vi "main.vi"() -> ()   [LabVIEW 2014]
uses:
  E:/labview_all/LabVIEW 2014/examples/Design Patterns/State Machine/support/State Machine Fundamentals - State Enum.ctl
  <vilib>/myRIO/Common/Instrument Driver Framework/myRIO v1.0/UART/vis/myRIO v1.0 Close UART.vi
  <vilib>/myRIO/Common/Instrument Driver Framework/Utilities/vis/FPGA Ref Manager.vi
  <vilib>/myRIO/Common/Instrument Driver Framework/myRIO v1.0/myRIO v1.0 Reset FPGA.vi
  <vilib>/myRIO/Common/Instrument Driver Framework/myRIO v1.0/IRQ/vis/myRIO v1.0 IRQ Info FGV.vi
  <vilib>/myRIO/Common/Instrument Driver Framework/myRIO v1.0/IRQ/vis/myRIO v1.0 Timer IRQ Info FGV.vi
  <vilib>/myRIO/Common/Instrument Driver Framework/myRIO v1.0/IRQ/vis/myRIO v1.0 ISR Agent.vi
  <vilib>/myRIO/Instrument Drivers/Utilities/Utilities.lvlib
panel:
  in  "布尔":bool
  out "y1 2":i32
  out "y1":i32
  out "shuzhi":dbl
  out "shuiping":dbl
  out "采集速度":bool
  out "state":T1
  in  "车速控制":dbl(slide) scale=-1.0..1.0
  in  "舵机":dbl(slide) min=-100.0 max=100.0 scale=-200.0..200.0
  out "Right（0）":bool
  out "Left（1）":bool
  out "四个角点":i32[][](array[numeric])
  in  "停止":bool
  out "Image":T2(plugin-control)
  # "X"
  # "Y"
  # "X"
  # "Y"
  # "左下"
  # "左上"
  # "右下"
  # "右上"
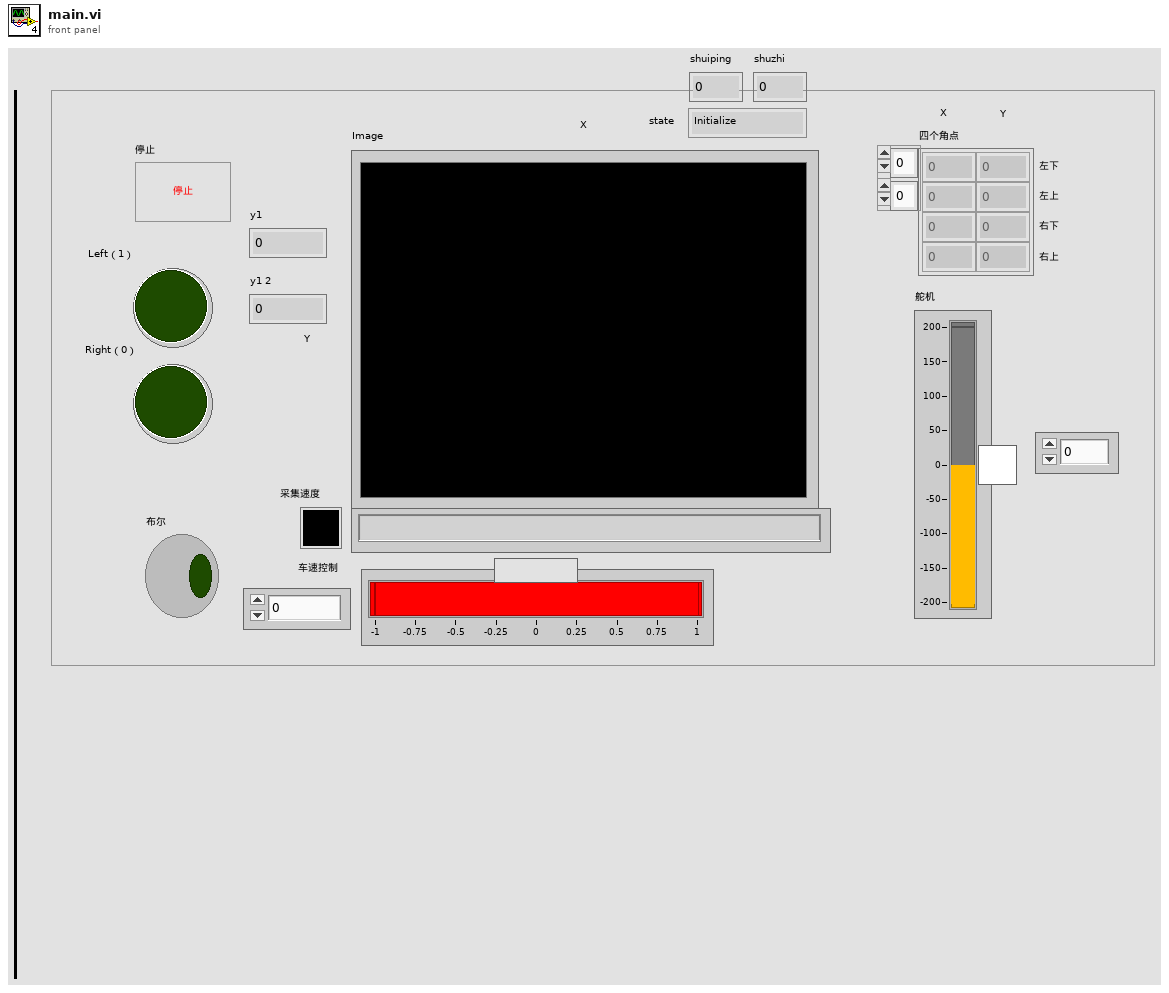
[diagram p1: front panel]
types:
  T1 = typedef "State Machine Fundamentals - State Enum.ctl" = enum16{"Initialize", "L or R", "L1", "L2", "R1", "R2", "IN", "STOP"}
  T2 = typedef "IMAQ Image.ctl" = refnum<image>
  T3 = cluster{"Optional Rectangle[0]":i32, "Optional Rectangle[1]":i32, "Optional Rectangle[2]":i32, "Optional Rectangle[3]":i32, "Optional Rectangle[4]":i32}
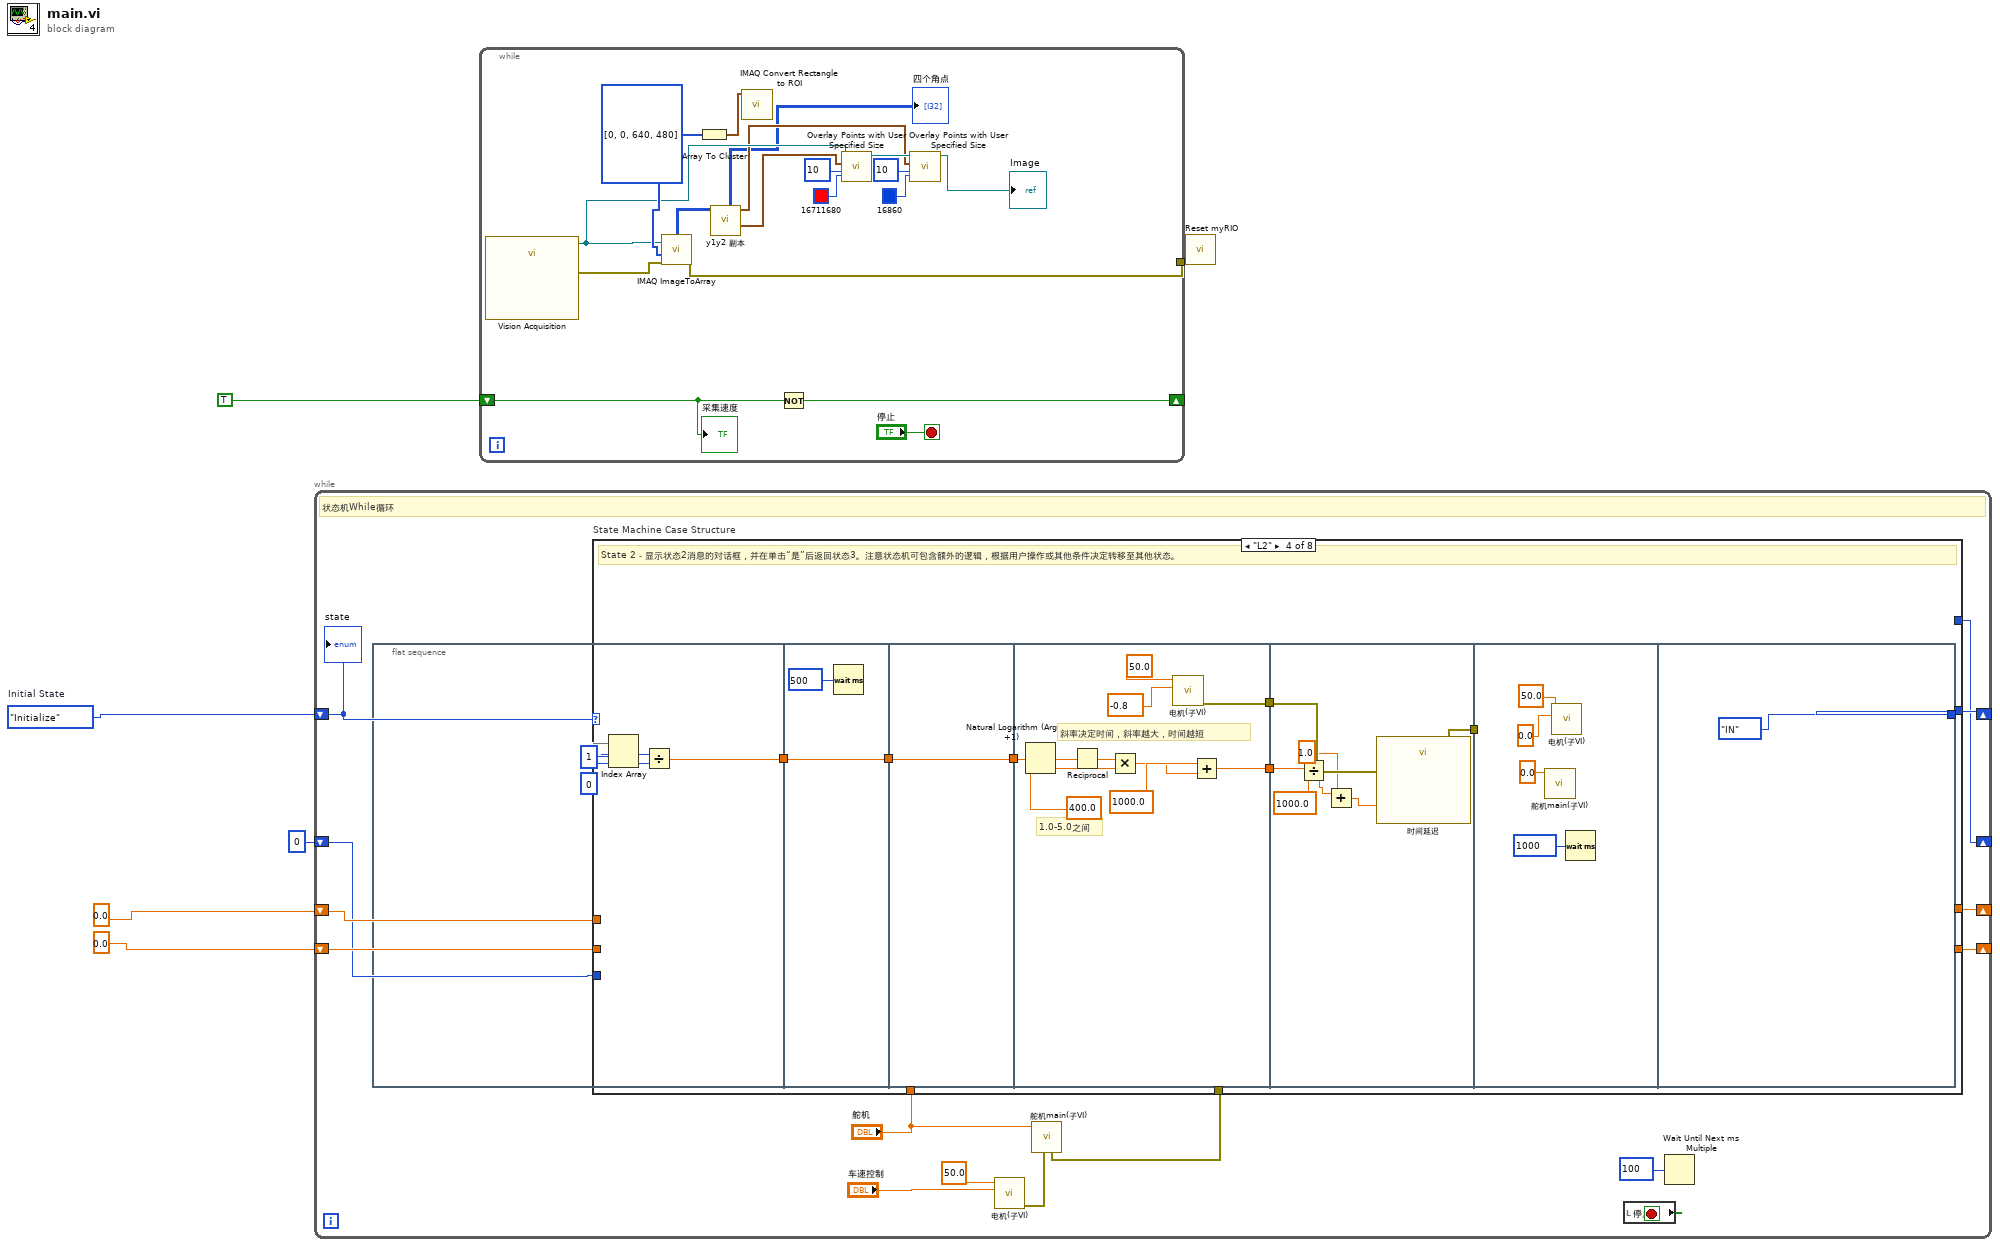
[diagram p0: block diagram]
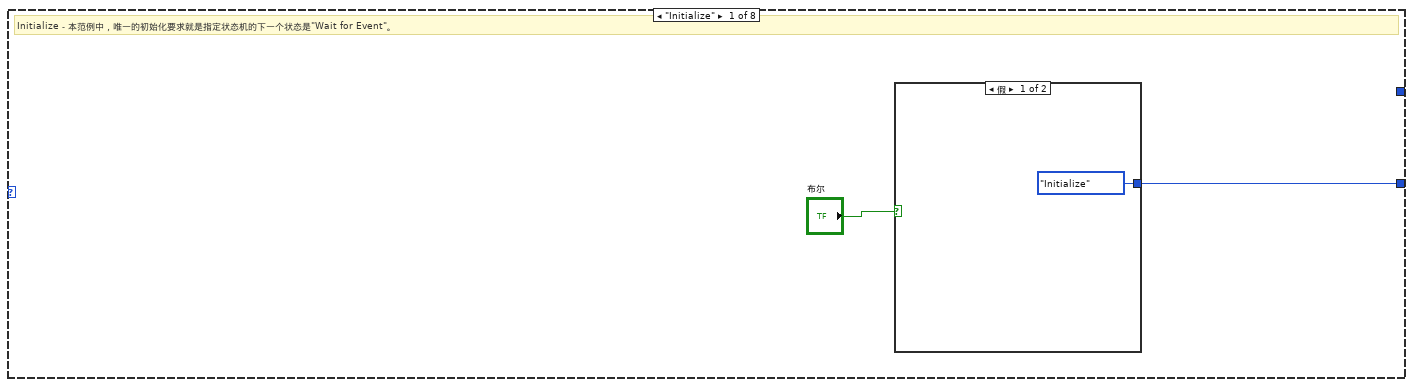
[diagram p2: hidden frame]
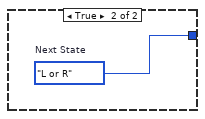
[diagram p3: hidden frame]
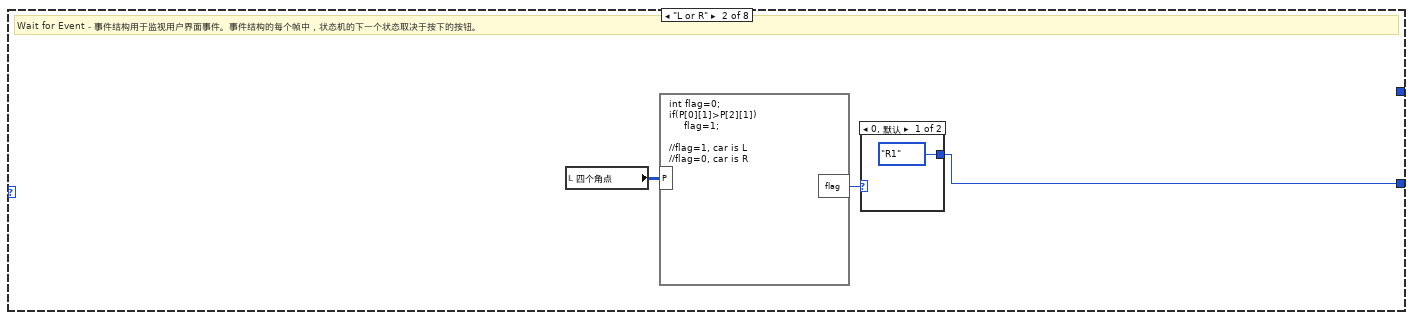
[diagram p4: hidden frame]
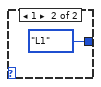
[diagram p5: hidden frame]
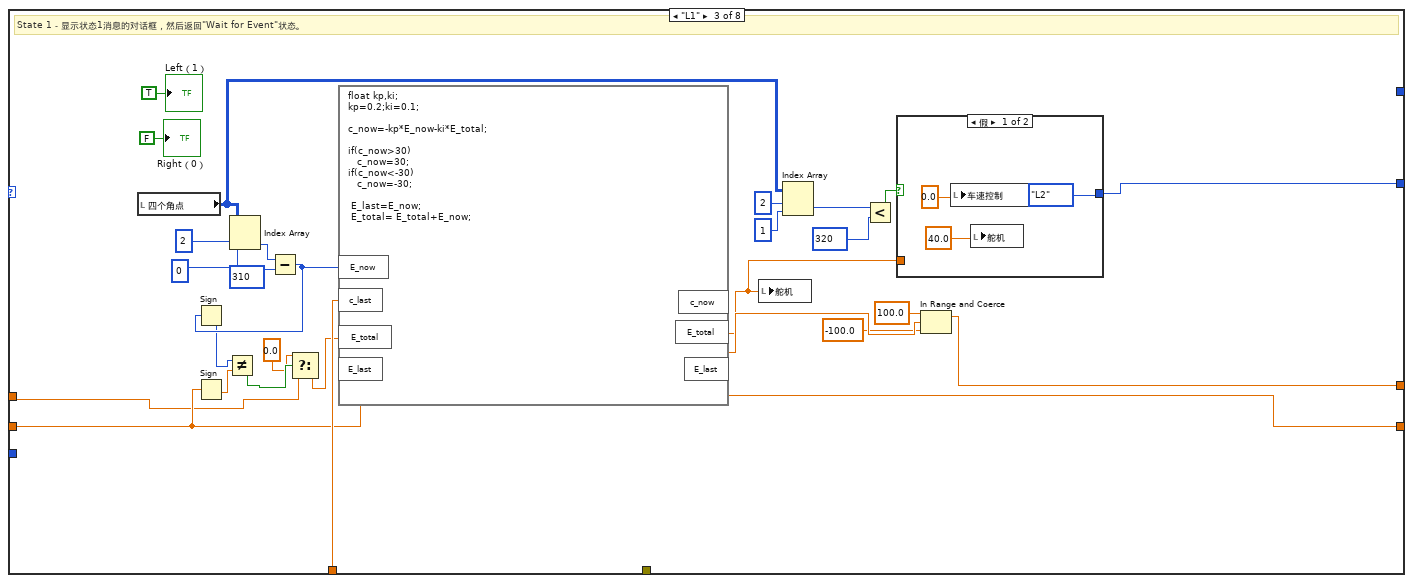
[diagram p6: hidden frame]
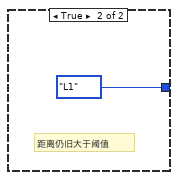
[diagram p7: hidden frame]
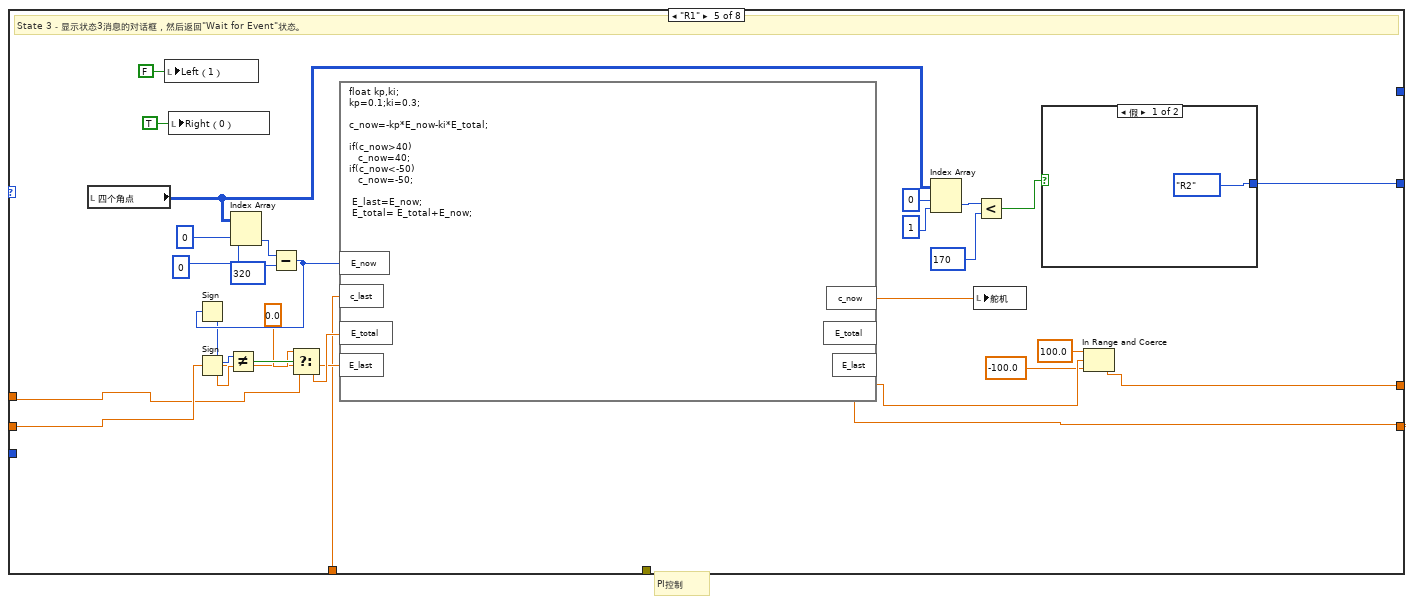
[diagram p8: hidden frame]
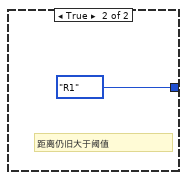
[diagram p9: hidden frame]
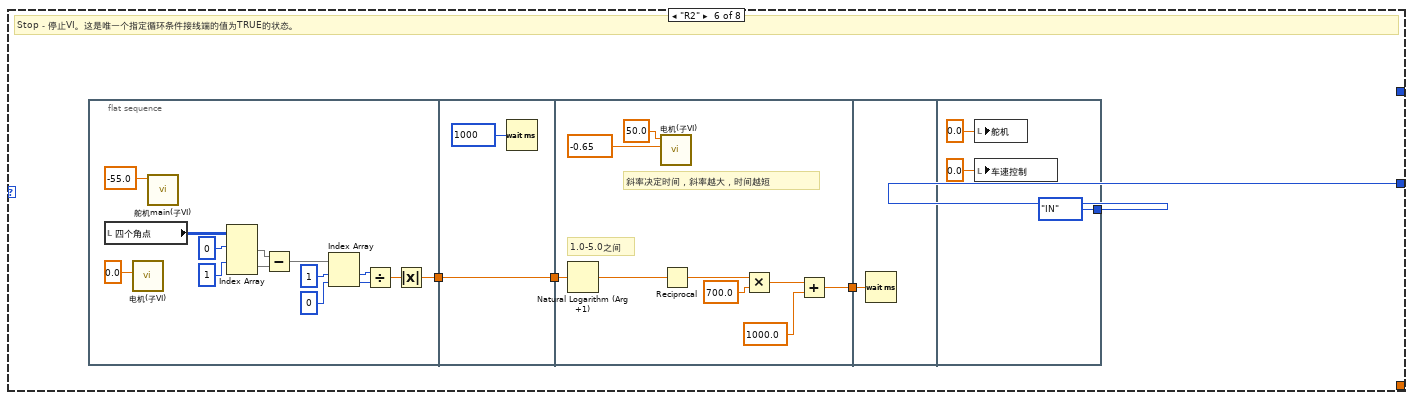
[diagram p10: hidden frame]
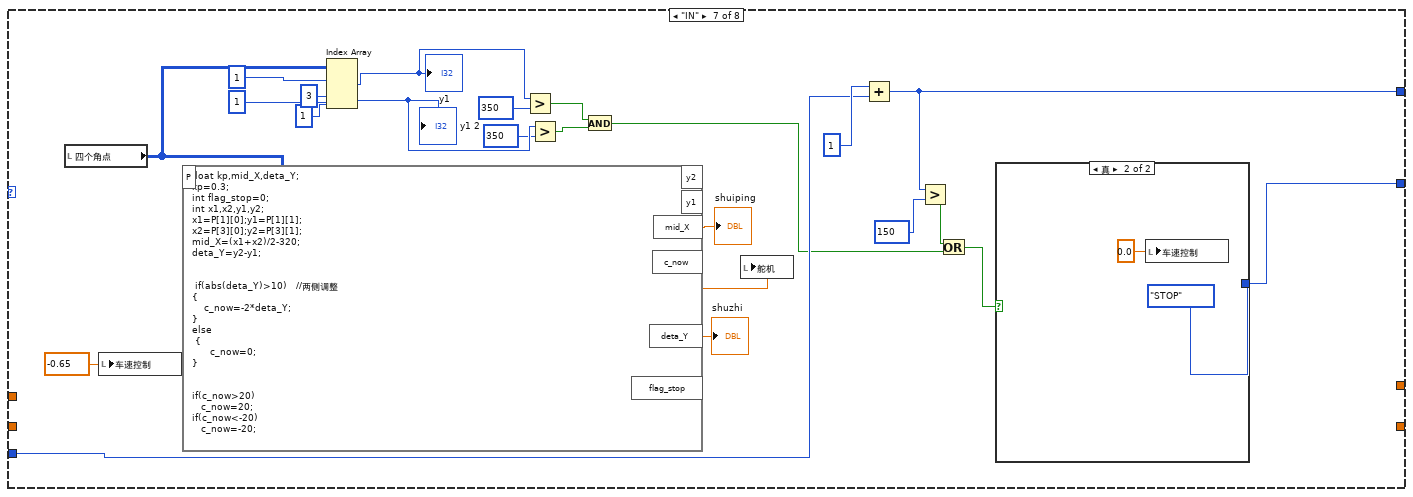
[diagram p11: hidden frame]
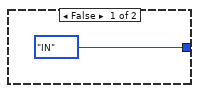
[diagram p12: hidden frame]
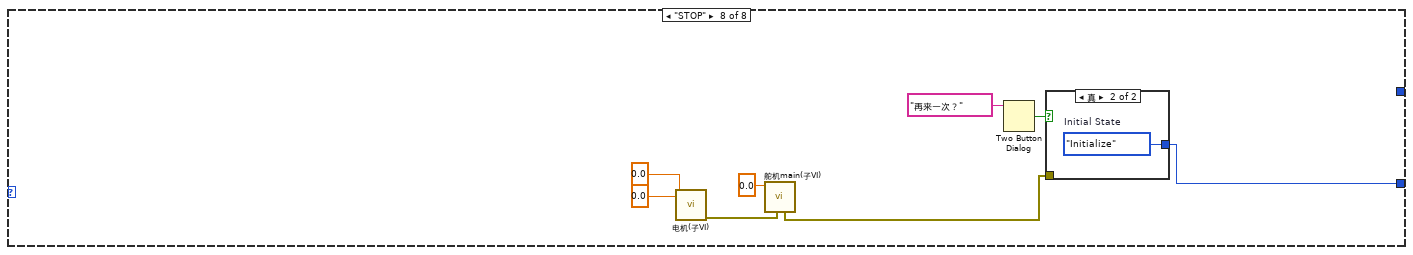
[diagram p13: hidden frame]
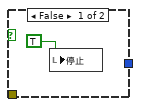
[diagram p14: hidden frame]
diagram:
  w4 = State_Machine_Fundamentals_-_State_Enum."Initialize"  # Initial State
  n1 = while {
    shift-right: [w20] -> _
    shift-left: 0.0 -> [w21]
    shift-right: [w16] -> _
    shift-left: 0.0 ("E_next") -> [w15]
    shift-right: [w11] -> _
    shift-left: w4 -> [w12]
    shift-right: [w8] -> _
    shift-left: 0 -> [w7]
    stop <- w9 stop-if-true
    # "状态机While循环"
    n2 = call "电机(子VI).vi"("车速控制"="车速控制", "hz"=50.0) -> ("错误输出"=w10:errorcluster)  [unwired: 9 in]
    n3 = call "舵机main(子VI).vi"("error in (no error)"=w10, "舵机"="舵机") -> ("error out"=w13:errorcluster)  [unwired: 9 in]
    n4 = case "State Machine Case Structure" shown="\"L2\"" w12 {
      tunnel: w21 -> [_ _ w44 _ w113 _ _ _]
      tunnel: [_ _ w41 _ w111 _ _ _] -> w20
      tunnel: "舵机" -> [_ _ w52 _ w110 _ _ _]
      tunnel: [_ _ w51 _ w112 _ _ _] -> w16
      tunnel: w15 -> [_ _ w49 _ w114 _ _ _]
      tunnel: w13 -> [_ _ _ _ _ _ _ _]
      tunnel: [w23 w27 w33 w67 w108 w136 w190 w202] -> w11
      tunnel: [_ _ _ _ _ _ w183 _] -> w8
      tunnel: w7 -> [_ _ _ _ _ _ w182 _]
      frame "Initialize" {
        # "Initialize－本范例中，唯一的初始化要求就是指定状态机的下一个状态是\"Wait for Event\"。"
        n5 = case shown="假" "布尔" {
          tunnel: [State_Machine_Fundamentals_-_State_Enum."Initialize" ("Next State") w25] -> w23
          frame False {
          }
          frame True {
            w25 = State_Machine_Fundamentals_-_State_Enum."L or R"  # Next State
          }
        }
      }
      frame "L or R" {
        # "Wait for Event－事件结构用于监视用户界面事件。事件结构的每个帧中，状态机的下一个状态取决于按下的按钮。"
        n6 = local read "四个角点"() -> (w26:i32[][])
        n7 = formula code="int flag=0;\nif(P[0][1]>P[2][1])\n     flag=1;\n\n//flag=1, car is L\n//flag=0, car is R"("P"=w26) -> ("flag"=w28:i32)
        n8 = case shown="0, 默认" w28 {
          tunnel: [State_Machine_Fundamentals_-_State_Enum."R1" State_Machine_Fundamentals_-_State_Enum."L1"] -> w27
          frame 0, Default {
          }
          frame 1 {
          }
        }
      }
      frame "L1" {
        # "PI控制"
        # "State 1－显示状态1消息的对话框，然后返回\"Wait for Event\"状态。"
        n9 = local read "四个角点"() -> (w38:i32[][])
        n10 = Sign(1:w49) -> (0:w47:dbl)
        n11 = Index Array(array=w38, index (row)=2 ("索引 (行)"), index (col)=0 ("禁用的索引 (列)")) -> (element=w54:i32)
        n12 = Subtract(x=w54, y=310) -> (x-y=w50:i32)
        n13 = Sign(1:w50) -> (0:w48:i32)
        n14 = Not Equal?(x=w48, y=w47) -> (x != y?=w45:bool)
        n15 = Select(t=0.0, s=w45, f=w44) -> (s? t:f=w46:dbl)
        n16 = formula code="float kp,ki;\nkp=0.2;ki=0.1;\n\nc_now=-kp*E_now-ki*E_total;\n\nif(c_now>30)\n   c_now=30;\nif(c_now<-30)\n   c_now=-30;\n\n E_last=E_now;\n E_total= E_total+E_now;"("E_now"=w50, "c_last"=w52, "E_total"=w46, "E_last"=w49) -> ("c_now"=w32:dbl, "E_total"=w42:dbl, "E_last"=w51:dbl)
        n17 = local write "舵机"(w32) -> ()
        n18 = Index Array(array=w38, index (row)=2 ("索引 (行)"), index (col)=1 ("禁用的索引 (列)")) -> (element=w35:i32)
        n19 = Less?(x=w35, y=320) -> (x < y?=w34:bool)
        n20 = case shown="假" w34 {
          tunnel: [State_Machine_Fundamentals_-_State_Enum."L2" State_Machine_Fundamentals_-_State_Enum."L1"] -> w33
          tunnel: w32 -> [_ _]
          frame False {
            n21 = local write "车速控制"(0.0 ("舵机")) -> ()
            n22 = local write "舵机"(40.0 ("舵机")) -> ()
          }
          frame True {
            # "距离仍旧大于阈值"
          }
        }
        n23 = In Range and Coerce(upper limit=100.0 ("上限"), x=w42, lower limit=-100.0 ("上限")) -> (coerced(x)=w41:dbl)  [unwired: 1 out]
        "Left（1）" <- TRUE ("Right（0） or Left（1）?")
        "Right（0）" <- FALSE ("Right（0） or Left（1）?")
      }
      frame "L2" {
        # "State 2－显示状态2消息的对话框，并在单击“是”后返回状态3。注意状态机可包含额外的逻辑，根据用户操作或其他条件决定转移至其他状态。"
        n24 = flat-sequence {
          tunnel: [w70] -> w69
          tunnel: [w81] -> w66
          tunnel: w69 -> [w81]
          tunnel: w66 -> [w83]
          tunnel: [w83] -> w65
          tunnel: w65 -> [w92]
          tunnel: [w89] -> w68
          tunnel: [w84] -> w64
          tunnel: w68 -> [w98]
          tunnel: w64 -> [w100]
          tunnel: [w99] -> w63
          tunnel: w63 -> [_]
          tunnel: [State_Machine_Fundamentals_-_State_Enum."IN"] -> w67
          frame #0 {
            n25 = local read "四个角点"() -> (w80:i32[][])
            n26 = Index Array(array=w80, index (row) #1=2 ("索引 (行)"), index (row) #2=3 ("索引 (行)")) -> (element #1=w77:i32[], element #2=w76:i32[])  [unwired: 2 in]
            n27 = Subtract(x=w77, y=w76) -> (x-y=w75:i32[])
            n28 = Index Array(array=w75, index #1=1 ("索引"), index #2=0 ("索引")) -> (element #1=w72:i32, element #2=w71:i32)
            n29 = Divide(x=w72, y=w71) -> (x/y=w70:dbl)
          }
          frame #1 {
            n30 = Wait (ms)(milliseconds to wait=u32 500 ("等待时间（毫秒）")) -> ()  [unwired: 1 out]
          }
          frame #2 {
          }
          frame #3 {
            # "1.0-5.0之间"
            # "斜率决定时间，斜率越大，时间越短"
            n31 = Natural Logarithm (Arg +1)(1:w92) -> (0:w88:dbl)
            n32 = Reciprocal(x=w88) -> (1/x=w87:dbl)
            n33 = Multiply(x=w87, y=400.0) -> (x*y=w86:dbl)
            n34 = call "电机(子VI).vi"("车速控制"=-0.8, "hz"=50.0) -> ("错误输出"=w84:errorcluster)  [unwired: 9 in]
            n35 = Add(x=1000.0 ("y"), y=w86) -> (x+y=w89:dbl)
          }
          frame #4 {
            n36 = Divide(x=w98, y=1000.0) -> (x/y=w95:dbl)
            n37 = Add(x=w95, y=1.0) -> (x+y=w96:dbl)
            n38 = call "时间延迟"("error in (no error)"=w100, "Delay Time (s)"=w96) -> ("error out"=w99:errorcluster)  [unwired: 9 in]
          }
          frame #5 {
            n39 = call "舵机main(子VI).vi"("舵机"=0.0) -> ()  [unwired: 10 in, 1 out]
            n40 = call "电机(子VI).vi"("车速控制"=0.0, "hz"=50.0) -> ()  [unwired: 9 in, 1 out]
            n41 = Wait (ms)(milliseconds to wait=u32 1000 ("等待时间（毫秒）")) -> ()  [unwired: 1 out]
          }
          frame #6 {
          }
        }
      }
      frame "R1" {
        # "PI控制"
        # "State 3－显示状态3消息的对话框，然后返回\"Wait for Event\"状态。"
        n42 = local read "四个角点"() -> (w106:i32[][])
        n43 = local write "Left（1）"(FALSE ("Right（0） or Left（1）?")) -> ()
        n44 = local write "Right（0）"(TRUE ("Right（0）")) -> ()
        n45 = Sign(1:w114) -> (0:w125:dbl)
        n46 = Index Array(array=w106, index (row)=0 ("索引 (行)"), index (col)=0 ("禁用的索引 (列)")) -> (element=w129:i32)
        n47 = Subtract(x=w129, y=320) -> (x-y=w127:i32)
        n48 = Sign(1:w127) -> (0:w126:i32)
        n49 = Not Equal?(x=w126, y=w125) -> (x != y?=w123:bool)
        n50 = Select(t=0.0, s=w123, f=w113) -> (s? t:f=w124:dbl)
        n51 = formula code="float kp,ki;\nkp=0.1;ki=0.3;\n\nc_now=-kp*E_now-ki*E_total;\n\nif(c_now>40)\n   c_now=40;\nif(c_now<-50)\n   c_now=-50;\n\n E_last=E_now;\n E_total= E_total+E_now;"("E_now"=w127, "c_last"=w110, "E_total"=w124, "E_last"=w114) -> ("c_now"=w109:dbl, "E_total"=w121:dbl, "E_last"=w112:dbl)
        n52 = Index Array(array=w106, index (row)=0 ("索引 (行)"), index (col)=1 ("禁用的索引 (列)")) -> (element=w117:i32)
        n53 = local write "舵机"(w109) -> ()
        n54 = Less?(x=w117, y=170) -> (x < y?=w116:bool)
        n55 = case shown="假" w116 {
          tunnel: [State_Machine_Fundamentals_-_State_Enum."R2" State_Machine_Fundamentals_-_State_Enum."R1"] -> w108
          frame False {
          }
          frame True {
            # "距离仍旧大于阈值"
          }
        }
        n56 = In Range and Coerce(upper limit=100.0 ("上限"), x=w121, lower limit=-100.0 ("上限")) -> (coerced(x)=w111:dbl)  [unwired: 1 out]
      }
      frame "R2" {
        # "Stop－停止VI。这是唯一个指定循环条件接线端的值为TRUE的状态。"
        n57 = flat-sequence {
          tunnel: [w140] -> w139
          tunnel: [w154] -> w138
          tunnel: w139 -> [w154]
          tunnel: w138 -> [w163]
          tunnel: [w160] -> w137
          tunnel: w137 -> [w165]
          tunnel: [State_Machine_Fundamentals_-_State_Enum."IN"] -> w136
          frame #0 {
            n58 = local read "四个角点"() -> (w153:i32[][])
            n59 = call "电机(子VI).vi"("车速控制"=0.0) -> ()  [unwired: 10 in, 1 out]
            n60 = call "舵机main(子VI).vi"("舵机"=-55.0) -> ()  [unwired: 10 in, 1 out]
            n61 = Index Array(array=w153, index (row) #1=0 ("索引 (行)"), index (row) #2=1 ("索引 (行)")) -> (element #1=w150:i32[], element #2=w149:i32[])  [unwired: 2 in]
            n62 = Subtract(x=w150, y=w149) -> (x-y=w148:i32[])
            n63 = Index Array(array=w148, index #1=1 ("索引"), index #2=0 ("索引")) -> (element #1=w145:i32, element #2=w144:i32)
            n64 = Divide(x=w145, y=w144) -> (x/y=w141:dbl)
            n65 = Absolute Value(x=w141) -> (abs(x)=w140:dbl)
          }
          frame #1 {
            n66 = Wait (ms)(milliseconds to wait=u32 1000 ("等待时间（毫秒）")) -> ()  [unwired: 1 out]
          }
          frame #2 {
            # "1.0-5.0之间"
            # "斜率决定时间，斜率越大，时间越短"
            n67 = Natural Logarithm (Arg +1)(1:w163) -> (0:w159:dbl)
            n68 = call "电机(子VI).vi"("车速控制"=-0.65, "hz"=50.0) -> ()  [unwired: 9 in, 1 out]
            n69 = Reciprocal(x=w159) -> (1/x=w158:dbl)
            n70 = Multiply(x=w158, y=700.0) -> (x*y=w157:dbl)
            n71 = Add(x=w157, y=1000.0) -> (x+y=w160:dbl)
          }
          frame #3 {
            n72 = Wait (ms)(milliseconds to wait=w165) -> ()  [unwired: 1 out]
          }
          frame #4 {
            n73 = local write "舵机"(0.0 ("舵机")) -> ()
            n74 = local write "车速控制"(0.0 ("车速控制")) -> ()
          }
        }
      }
      frame "IN" {
        n75 = local read "四个角点"() -> (w181:i32[][])
        n76 = local write "车速控制"(-0.65 ("车速控制")) -> ()
        n77 = formula code="float kp,mid_X,deta_Y;\nkp=0.3;\nint flag_stop=0;\nint x1,x2,y1,y2;\nx1=P[1][0];y1=P[1][1];\nx2=P[3][0];y2=P[3][1];\nmid_X=(x1+x2)/2-320;\ndeta_Y=y2-y1;\n\n\n if(abs(deta_Y)>10)   //两侧调整\n{\n    c_now=-2*deta_Y;\n}\nelse\n {   \n      c_now=0;\n}\n\n\nif(c_now>20)\n   c_now=20;\nif(c_now<-20)\n   c_now=-20;"("P"=w181) -> ("c_now"=w191:dbl, "mid_X"=→"shuiping":dbl, "deta_Y"=→"shuzhi":dbl)  [unwired: 3 out]
        n78 = Index Array(array=w181, index (row) #1=1 ("索引 (行)"), index (col) #1=1 ("禁用的索引 (列)"), index (row) #2=3 ("索引 (行)"), index (col) #2=1 ("禁用的索引 (列)")) -> (element #1=w176:i32, element #2=w175:i32)
        "y1" <- w176
        "y1 2" <- w175
        n79 = Greater?(x=w176, y=350) -> (0:w172:bool)
        n80 = Greater?(x=w175, y=350) -> (0:w171:bool)
        n81 = And(x=w172, y=w171) -> (x .and. y?=w170:bool)
        n82 = local write "舵机"(w191) -> ()
        n83 = Add(x=1, y=w182) -> (x+y=w183:i32)
        n84 = Greater?(x=w183, y=150) -> (0:w185:bool)
        n85 = Or(x=w185, y=w170) -> (x .or. y?=w184:bool)
        n86 = case shown="真" w184 {
          tunnel: [State_Machine_Fundamentals_-_State_Enum."IN" State_Machine_Fundamentals_-_State_Enum."STOP"] -> w190
          frame False {
          }
          frame True {
            n87 = local write "车速控制"(0.0 ("车速控制")) -> ()
          }
        }
      }
      frame "STOP" {
        n88 = call "电机(子VI).vi"("车速控制"=0.0, "hz"=0.0) -> ("错误输出"=w196:errorcluster)  [unwired: 9 in]
        n89 = call "舵机main(子VI).vi"("error in (no error)"=w196, "舵机"=0.0) -> ("error out"=w195:errorcluster)  [unwired: 9 in]
        n90 = Two Button Dialog(message="再来一次？" ("消息")) -> (T button?=w201:bool)  [unwired: 2 in]
        n91 = case shown="真" w201 {
          tunnel: [_ w204] -> w202
          tunnel: w195 -> [_ _]
          frame False {
            n92 = local write "停止"(TRUE ("停止")) -> ()
          }
          frame True {
            w204 = State_Machine_Fundamentals_-_State_Enum."Initialize"  # Initial State
          }
        }
      }
    }
    n93 = local read "停止"() -> (w9:bool)
    n94 = Wait Until Next ms Multiple(millisecond multiple=u32 100 ("毫秒倍数")) -> ()  [unwired: 1 out]
    "state" <- w12
  }
  n95 = while {
    tunnel: [w217] -> w2
    shift-right: [w213] -> _
    shift-left: TRUE -> [w212]
    stop <- "停止" stop-if-true
    w219 = i32[] [0, 0, 640, 480] ("Optional Rectangle")
    n96 = call "Vision Acquisition"() -> ("Image Out"=w214:T2, "error out"=w218:errorcluster)  [unwired: 26 in]
    n97 = call "IMAQ ImageToArray"("error in (no error)"=w218, "Optional Rectangle"=w219, "Image"=w214) -> ("error out"=w217:errorcluster, "Image Pixels (U8)"=w220:u8[][])  [unwired: 1 in, 3 out]
    n98 = Array To Cluster(array=w219) -> (cluster=w221:T3)
    n99 = call "y1y2 副本.vi"("Image Pixels (U8)输入"=w220) -> ("right"=w211:cluster{i32, i32}[], "left"=w206:cluster{i32, i32}[], "四个角点"=→"四个角点":i32[][])  [unwired: 4 in, 2 out]
    n100 = call "IMAQ Convert Rectangle to ROI"("Rectangle"=w221) -> ()  [unwired: 8 in, 2 out]
    n101 = Not(x=w212) -> (.not. x?=w213:bool)
    n102 = call "Overlay Points with User Specified Size.vi"("Color"=u32 16711680, "Point Diameter (5)"=u32 10, "Points"=w211, "Image In"=w214) -> ("Image Out"=w210:T2)  [unwired: 6 in, 1 out]
    n103 = call "Overlay Points with User Specified Size.vi"("Color"=u32 16860, "Point Diameter (5)"=u32 10, "Points"=w206, "Image In"=w210) -> ("Image Out"=→"Image":T2)  [unwired: 6 in, 1 out]
    "采集速度" <- w212
  }
  n104 = call <vilib>:"Reset myRIO.vi"("error in (no error)"=w2) -> ()  [unwired: 10 in, 1 out]
